vi "create_random_image.vi"(8 "error in (no error)":errorcluster, 10 "array size":i32=128, 11 "ColorOverlay in":refnum<class "ColorOverlay.lvclass">) -> (0 "error out":errorcluster, 2 "random image out":T1(plugin-control), 3 "ColorOverlay out":refnum<class "ColorOverlay.lvclass">)   [LabVIEW 2010, in "ColorOverlay.lvclass"]
uses:
  ColorOverlay.lvclass
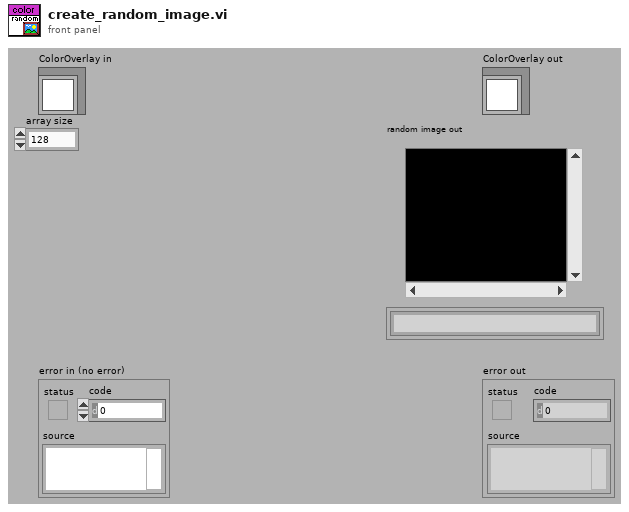
[diagram p1: front panel]
types:
  T1 = typedef "IMAQ Image.ctl" = refnum<image>
  T2 = typedef "Image Type" = u32
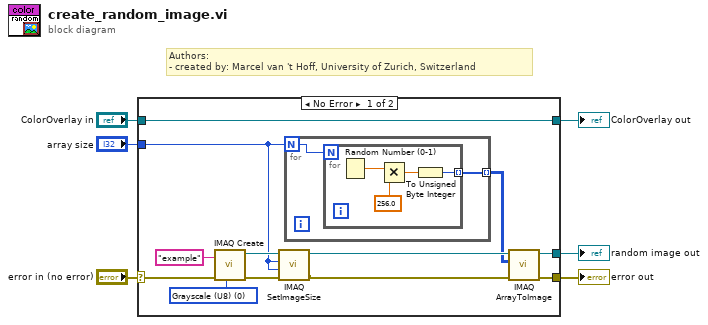
[diagram p0: block diagram]
diagram:
  # "Authors: \n- created by: Marcel van 't Hoff, University of Zurich, Switzerland"
  n1 = case shown="No Error" "error in (no error)" {
    selector: "error in (no error)" -> [w8 w26]
    tunnel: [w12 _] -> w1
    tunnel: "array size" -> [w10 _]
    tunnel: [w9 w26] -> w2
    tunnel: [w7 w25] -> w5
    tunnel: "ColorOverlay in" -> [w7 w25]
    frame No Error {
      w17 = T2 0 items=["Grayscale (U8)", "Grayscale (I16)", "Grayscale (SGL)", "Complex (CSG)", "RGB (U32)", "HSL (U32)", "RGB (U64)", "Grayscale (U16)"] ("Image Type")
      n2 = call "IMAQ Create"("Image Name"="example", "Image Type"=w17, "error in (no error)"=w8) -> ("New Image"=w15:T1, "error out"=w16:errorcluster)  [unwired: 2 in]
      n3 = call "IMAQ SetImageSize"("error in (no error)"=w16, "Y Resolution"=w10, "X Resolution"=w10, "Image"=w15) -> ("error out"=w13:errorcluster, "Image Out"=w14:T1)  [unwired: 1 in]
      n4 = for {
        N: w10 -> [w20]
        tunnel: [w19] -> w11 mode=indexing
        n5 = for {
          N: w20 -> [_]
          tunnel: [w21] -> w19 mode=indexing
          n6 = Random Number (0-1)() -> (number: 0 to 1=w24:dbl)
          n7 = Multiply(x=w24, y=256.0) -> (x*y=w22:dbl)
          n8 = To Unsigned Byte Integer(number=w22) -> (unsigned 8bit integer=w21:u8)
        }
      }
      n9 = call "IMAQ ArrayToImage"("error in (no error)"=w13, "Image Pixels (U8)"=w11, "Image"=w14) -> ("error out"=w9:errorcluster, "Image Out"=w12:T1)  [unwired: 7 in]
    }
    frame Error {
    }
  }
  "error out" <- w2
  "ColorOverlay out" <- w5
  "random image out" <- w1
